vi "Write Vector Signal Generator.lvclass.vi"(10 "Vector Signal Generator.lvclass":refnum<class "Vector Signal Generator.lvclass">, 11 "MCCW ACLR in":refnum<class "MCCW ACLR.lvclass">) -> (3 "MCCW ACLR out":refnum<class "MCCW ACLR.lvclass">)   [LabVIEW 2020, in "MCCW ACLR.lvclass"]
uses:
  MCCW ACLR.lvclass
  Instruments/Vector Signal Generator/Vector Signal Generator.lvclass
  MCCW ACLR.lvclass/MCCW ACLR.ctl
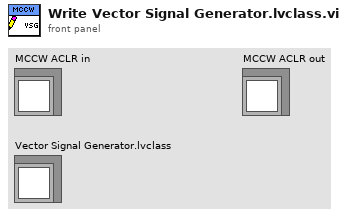
[diagram p1: front panel]
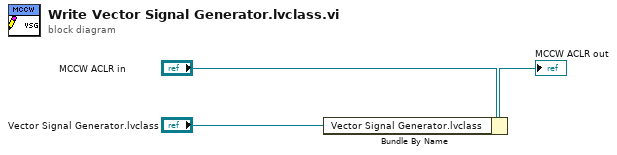
[diagram p0: block diagram]
diagram:
  n1 = Bundle By Name(cluster="MCCW ACLR in", "Vector Signal Generator.lvclass"="Vector Signal Generator.lvclass") -> (→"MCCW ACLR out":refnum<class "MCCW ACLR.lvclass">)
